vi "Set Trigger.vi"(8 "error in (no error)":errorcluster, 11 "CCDCamera in":refnum<class "Simulated_CCD_Camera.lvclass">) -> (0 "error out":errorcluster, 3 "CCDCamera out":refnum<class "Simulated_CCD_Camera.lvclass">)   [LabVIEW 2018, in "Simulated_CCD_Camera.lvclass"]
uses:
  Simulated_CCD_Camera.lvclass
  Simulated_CCD_Camera.lvclass/Simulated_CCD_Camera.ctl
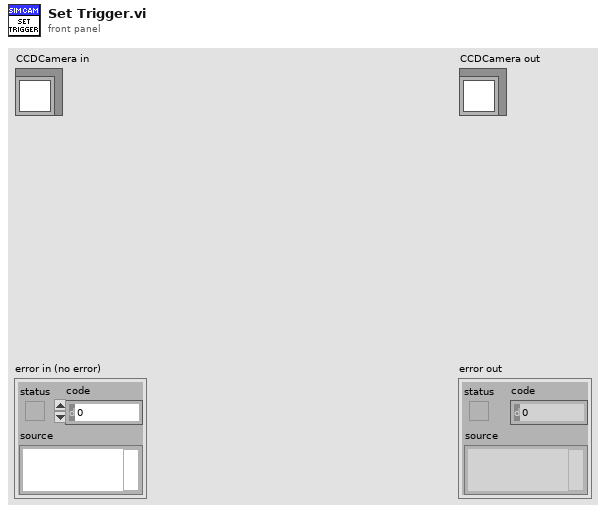
[diagram p1: front panel]
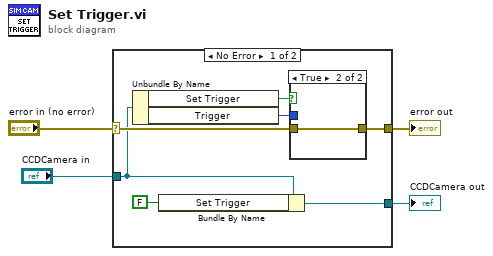
[diagram p0: block diagram]
diagram:
  n1 = case shown="No Error" "error in (no error)" {
    selector: "error in (no error)" -> [w10 w15]
    tunnel: [w11 w15] -> w3
    tunnel: [w6 w14] -> w1
    tunnel: "CCDCamera in" -> [w7 w14]
    frame No Error {
      n2 = Unbundle By Name(w7) -> ("Set Trigger"=w8:bool, "Trigger"=w9:u16)
      n3 = Bundle By Name(cluster=w7, "Set Trigger"=FALSE ("CCD Config.Set Trigger")) -> (w6:refnum<class "Simulated_CCD_Camera.lvclass">)
      n4 = case shown="True" w8 {
        tunnel: [w12 w13] -> w11
        tunnel: w10 -> [w12 w13]
        tunnel: w9 -> [_ _]
        frame False {
        }
        frame True {
        }
      }
    }
    frame Error {
    }
  }
  "error out" <- w3
  "CCDCamera out" <- w1
